vi "runHTSocketContact.vi"() -> ()   [LabVIEW 2012]
uses:
  <vilib>/Utility/file.llb/Read From Spreadsheet File (string).vi
  <vilib>/regexp/Match Regular Expression.xnode
panel:
  out "concatenated string 2":string
  in  "file path (dialog if empty)":path=path "C:/temp/ht/now/HTentity.txt"
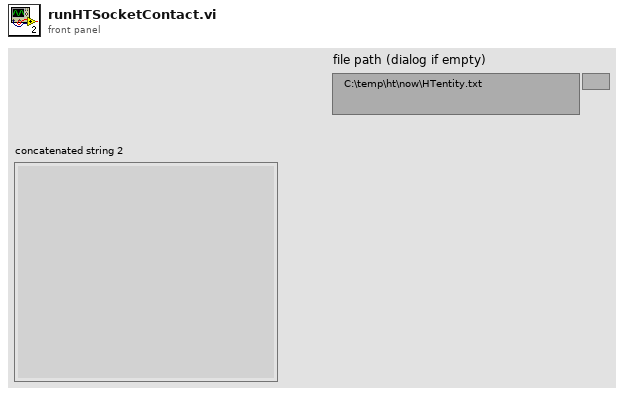
[diagram p1: front panel]
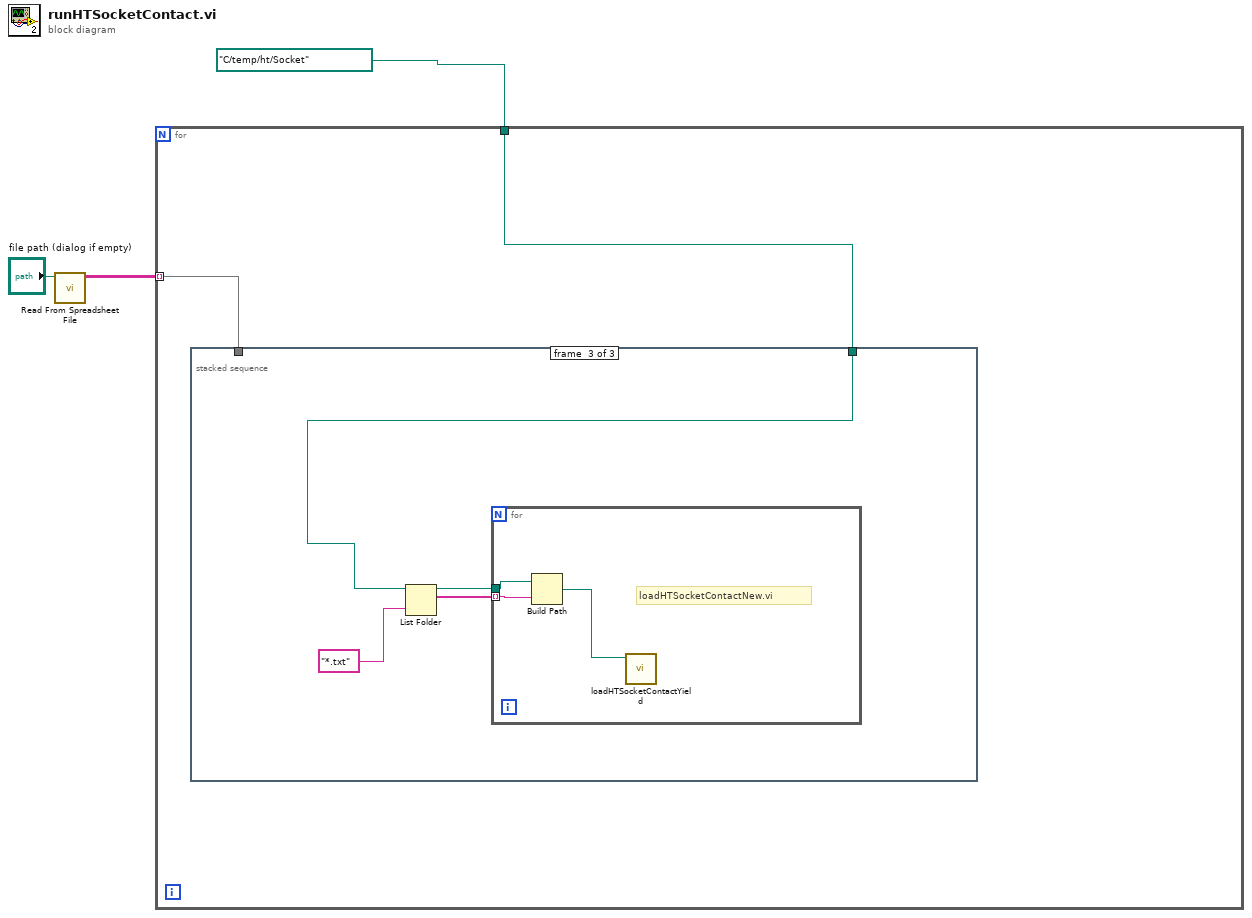
[diagram p0: block diagram]
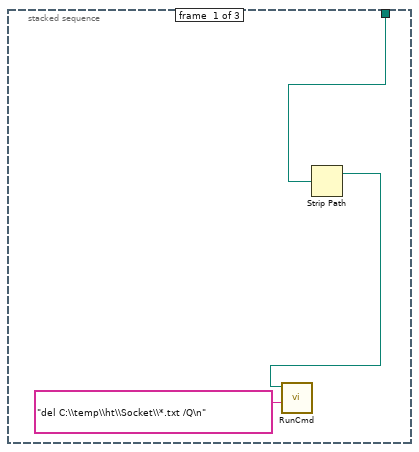
[diagram p2: hidden frame]
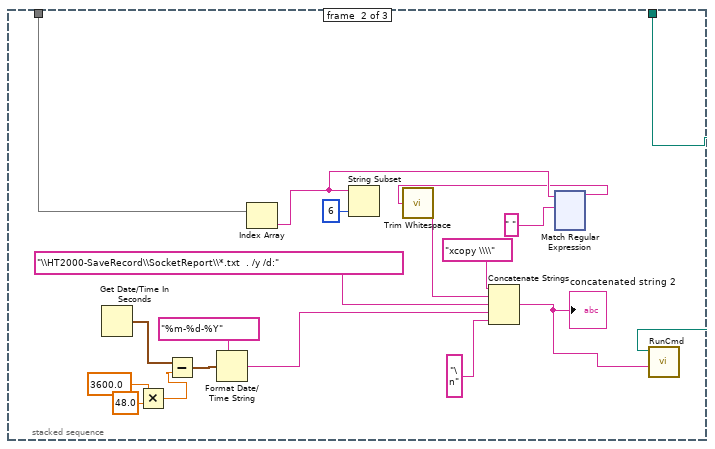
[diagram p3: hidden frame]
diagram:
  n1 = call-poly <vilib>:"Read From Spreadsheet File.vi"("file path (dialog if empty)"="file path (dialog if empty)") -> ("all rows"=w2:string[][])  [unwired: 6 in, 4 out]
  n2 = for {
    tunnel: w2 -> [w5] mode=indexing
    tunnel: path "C:/temp/ht/Socket" ("path") -> [w4]
    n3 = stacked-sequence {
      tunnel: w5 -> [_ w18 _]
      tunnel: w4 -> [w6 w9 w138]
      frame #0 {
        n4 = Strip Path(path=w6) -> (stripped path=w8:path)  [unwired: 1 out]
        n5 = call "RunCmd.vi"("Cmd String"="del C:\\temp\\ht\\Socket\\*.txt /Q\n", "working directory"=w8) -> ()  [unwired: 8 in, 2 out]
      }
      frame #1 {
        n6 = Get Date/Time In Seconds() -> (seconds since 1Jan1904=w12:timestamp)
        n7 = Multiply(x=3600.0, y=48.0) -> (x*y=w14:dbl)
        n8 = Subtract(x=w12, y=w14) -> (x-y=w15:timestamp)
        n9 = Format Date/Time String(time format string (%c)="%m-%d-%Y", seconds (now)=w15) -> (date/time string=w11:string)  [unwired: 1 in]
        n10 = Index Array(array=w18) -> (element=w22:string)  [unwired: 1 in]
        n11 = String Subset(string=w22, length (rest)=6 ("length (rest)")) -> ()  [unwired: 1 in, 1 out]
        n12 = xnode "Match Regular Expression"("input string"=w22, "regular expression"=" ") -> ("before match"=w21:string)  [unwired: 4 in, 4 out]
        n13 = call <vilib>:"Trim Whitespace.vi"("string"=w21) -> ("trimmed string"=w19:string)  [unwired: 1 in]
        n14 = Concatenate Strings("xcopy \\\\" ("string"), w19, "\\HT2000-SaveRecord\\SocketReport\\*.txt  . /y /d:" ("string"), w11, "\n" ("string")) -> (w25:string)
        "concatenated string 2" <- w25
        n15 = call "RunCmd.vi"("Cmd String"=w25, "working directory"=w9) -> ()  [unwired: 8 in, 2 out]
      }
      frame #2 {
        n16 = List Folder(path=w138, pattern="*.txt") -> (path out=w140:path, filenames=w139:string[])  [unwired: 2 in, 2 out]
        n17 = for {
          tunnel: w140 -> [w144]
          tunnel: w139 -> [w143] mode=indexing
          # "loadHTSocketContactNew.vi"
          n18 = Build Path(base path=w144, name or relative path=w143) -> (appended path=w142:path)
          n19 = call "loadHTSocketContactYield.vi"("file (use dialog)"=w142) -> ()  [unwired: 11 in]
        }
      }
    }
  }
